vi "Set Message Window Ref.vi"(0 "reference in":refnum<class "Generic Utilities.lvclass">, 5 "error in (no error)":errorcluster) -> (14 "reference out":refnum<class "Generic Utilities.lvclass">, 19 "error out":errorcluster)   [LabVIEW 2022 SP3, in "Generic Utilities.lvclass"]
uses:
  Generic Utilities.lvclass
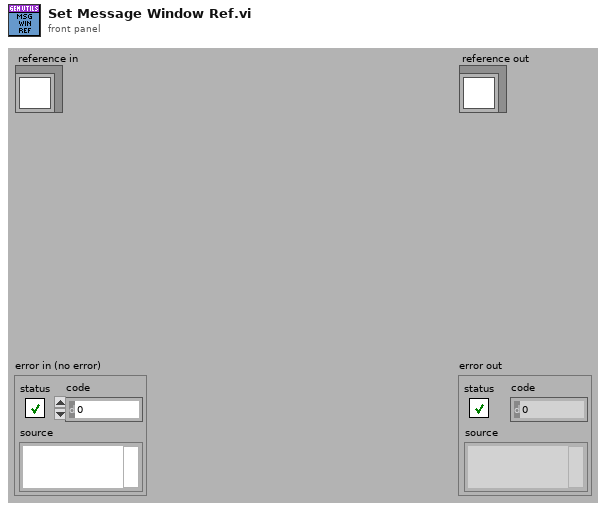
[diagram p1: front panel]
types:
  T1 = typedef "Generic Utilities.lvclass/ObjectAttributesRef.ctl" = refnum<data-value>
  T2 = typedef "Generic Utilities.lvclass/ObjectAttributes.ctl" = cluster{"GUI Parameters":T3, "State Machine Control":cluster{"Timeout":i32, "State Queue":string[], "State History":string[], "State History Length":i32}, "Logging File Path":path, "OBJ not a refnum?":bool, "Timer Start":timestamp, "FP Refnums":T4}
  T3 = typedef "Generic Utilities.lvclass/GUI Parameters.ctl" = cluster{"Application Name":string, "GUI VI Ref":refnum<vi>, "Close Panel?":bool, "Message Window ref":refnum<vi>, "Version #":string}
  T4 = typedef "Generic Utilities.lvclass/FP Refnums.ctl" = cluster{"Panel refnum":refnum<vi>, "Control Labels":string[], "Refnums":refnum<vi>[]}
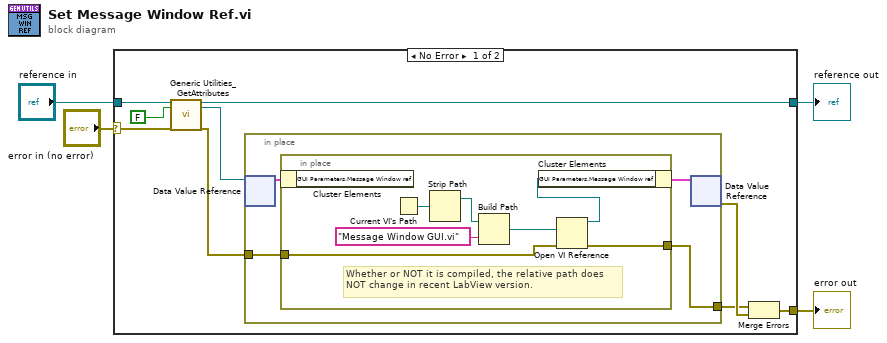
[diagram p0: block diagram]
diagram:
  n1 = case shown="No Error" "error in (no error)" {
    selector: "error in (no error)" -> [w8 w26]
    tunnel: [w13 w26] -> w3
    tunnel: [w7 w25] -> w1
    tunnel: "reference in" -> [w10 w25]
    frame No Error {
      n2 = call "Generic Utilities_GetAttributes.vi"("reference in"=w10, "return data? (T)"=FALSE, "error in (no error)"=w8) -> ("reference out"=w7:refnum<class "Generic Utilities.lvclass">, "attributes ref"=w6:T1, "error out"=w5:errorcluster)  [unwired: 13 in, 1 out]
      n3 = in-place {
        in-place-border: [w14] -> w11
        in-place-border: w5 -> [w15]
        n4 = in-place-dvr #1(w6) -> (w16:T2)  [unwired: 1 out]
        n5 = in-place {
          in-place-border: w15 -> [w19]
          in-place-border: [w18] -> w14
          # "Whether or NOT it is compiled, the relative path does NOT change in recent LabView version."
          n6 = in-place-cluster #2(w16) -> ()  [unwired: 1 out]
          n7 = Current VI's Path() -> (path=w23:path)
          n8 = Strip Path(path=w23) -> (stripped path=w21:path)  [unwired: 1 out]
          n9 = Build Path(base path=w21, name or relative path="Message Window GUI.vi") -> (appended path=w22:path)
          n10 = Open VI Reference(vi path=w22, error in (no error)=w19) -> (vi reference=w20:refnum<vi>, error out=w18:errorcluster)  [unwired: 4 in]
          n11 = in-place-cluster #2("GUI Parameters.Message Window ref"=w20) -> (w17:T2)
        }
        n12 = in-place-dvr #1(w17) -> (w12:errorcluster)  [unwired: 1 out]
      }
      n13 = Merge Errors(w11, w12) -> (w13:errorcluster)
    }
    frame Error {
    }
  }
  "error out" <- w3
  "reference out" <- w1
